vi "Get Network Adapter Settings.vi"(8 "error in":errorcluster, 11 "Refnum in":refnum<k21>) -> (0 "error out":errorcluster, 2 "Network Adapter Settings":T1[](array[typedef]) {"IP Address Request Mode" items=["Static"=1, "DHCP/Link Local"=2, "Link-Local Only"=4, "DHCP Only"=8]; "Adapter Type" items=["Ethernet"=1, "WLAN"=2]; "Adapter Mode" items=["Disabled"=1, "TCP/IP Ethernet"=2, "Deterministic"=4, "EtherCAT"=8, "TCP/IP WLAN Connect"=32, "TCP/IP WLAN Create"=64]}, 3 "Refnum out":refnum<k21>)   [LabVIEW 2015, in "RT Management.lvlib"]
uses:
  RT Management.lvlib
  Distributed Devices/Controls/NetworkAdapterSettings.ctl
  <vilib>/nisyscfg/Find Hardware.vi
  <vilib>/nisyscfg/Close (Hardware).vi
  <vilib>/nisyscfg/nisyscfg.lvlib
  <resource>/objmgr/niflexriosae.rc
  Distributed Devices/Device.lvclass
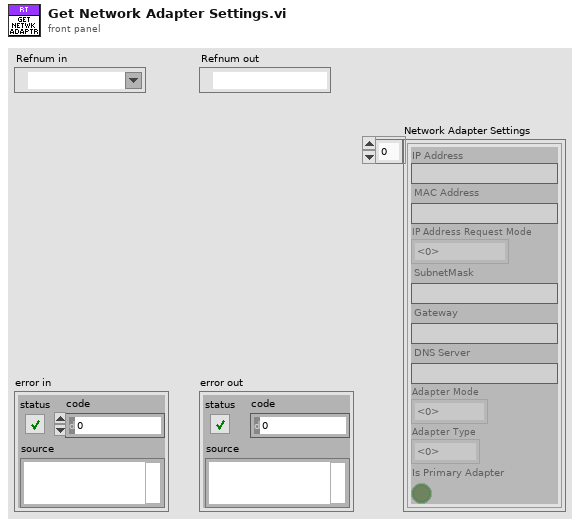
[diagram p1: front panel]
types:
  T1 = typedef "RT Management.lvlib/Device.lvclass/NetworkAdapterSettings.ctl" = cluster{"IP Address":string, "MAC Address":string, "IP Address Request Mode":u32, "SubnetMask":string, "Gateway":string, "DNS Server":string, "Adapter Mode":u32, "Adapter Type":u32, "Is Primary Adapter":bool}
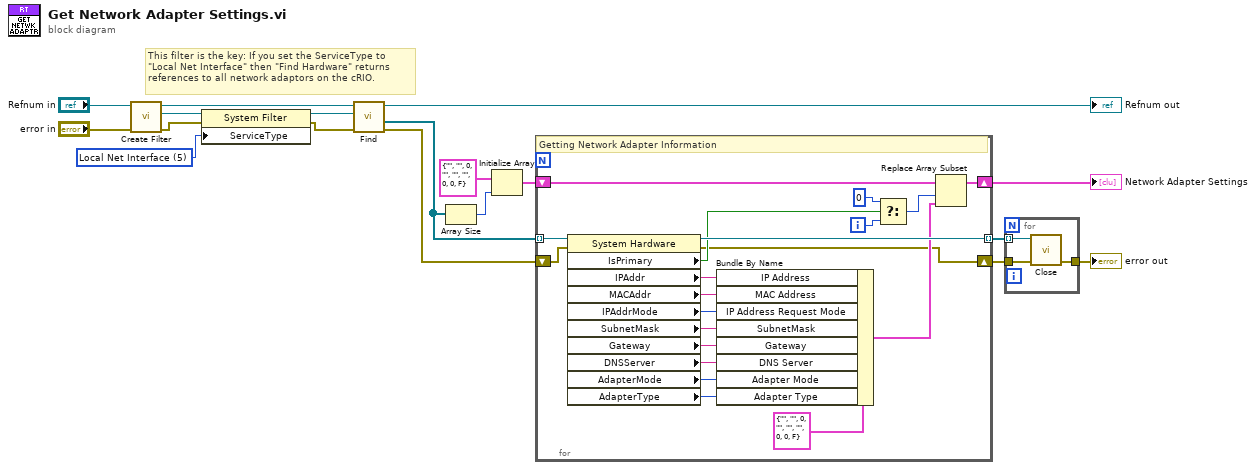
[diagram p0: block diagram]
diagram:
  w10 = u32 5 items=["NI Network Resource", "NI Real-Time", "NI System Configuration", "NI Web Interface", "Local System", "Local Net Interface", "Local Time Keeper", "Local Time Reference", "LXI Instrument"] ("Service Type")
  # "This filter is the key: If you set the ServiceType to\n\"Local Net Interface\" then \"Find Hardware\" returns\nreferences to all network adaptors on the cRIO."
  n1 = call <vilib>:"Create Filter.vi"("error in (no error)"="error in", "Session in"="Refnum in") -> ("error out"=w13:errorcluster, "Filter out"=w9:refnum<k20>, "Session out"=w8:refnum<k21>)  [unwired: 7 in]
  n2 = property class="System Filter"(reference=w9, error in=w13, "ServiceType"=w10) -> (reference out=w11:refnum<k20>, error out=w12:errorcluster)
  n3 = call-poly <vilib>:"Find.vi"("error in (no error)"=w12, "Filter in"=w11, "Session in"=w8) -> ("error out"=w14:errorcluster, "Resources out"=w4:refnum<k20>[], "Session out"=→"Refnum out":refnum<k21>)  [unwired: 5 in, 1 out]
  n4 = Array Size(array=w4) -> (size(s)=w3:i32)
  n5 = Initialize Array(T1 {"IP Address"="", "MAC Address"="", "IP Address Request Mode"=0, "SubnetMask"="", "Gateway"="", "DNS Server"="", "Adapter Mode"=0, "Adapter Type"=0, "Is Primary Adapter"=FALSE} ("Network Adapter Settings"), w3) -> (w1:T1[])
  n6 = for {
    tunnel: w4 -> [w37] mode=indexing
    shift-right: [w19] -> w17
    shift-left: w14 -> [w38]
    tunnel: [w32] -> w7 mode=indexing
    shift-right: [w20] -> w18
    shift-left: w1 -> [w26]
    i -> [w23]
    # "Getting Network Adapter Information"
    n7 = property class="System Hardware"(reference=w37, error in=w38) -> (reference out=w32:refnum<k20>, error out=w19:errorcluster, "IsPrimary"=w25:bool, "IPAddr"=w27:string, "MACAddr"=w33:string, "IPAddrMode"=w30:u32, "SubnetMask"=w34:string, "Gateway"=w35:string, "DNSServer"=w36:string, "AdapterMode"=w29:u32, "AdapterType"=w28:u32)
    n8 = Bundle By Name(cluster=T1 {"IP Address"="", "MAC Address"="", "IP Address Request Mode"=0, "SubnetMask"="", "Gateway"="", "DNS Server"="", "Adapter Mode"=0, "Adapter Type"=0, "Is Primary Adapter"=FALSE} ("Network Adapter Settings"), "IP Address"=w27, "MAC Address"=w33, "IP Address Request Mode"=w30, "SubnetMask"=w34, "Gateway"=w35, "DNS Server"=w36, "Adapter Mode"=w29, "Adapter Type"=w28) -> (w21:T1)
    n9 = Select(t=0 ("index"), s=w25, f=w23) -> (s? t:f=w22:i32)
    n10 = Replace Array Subset(array=w26, new element=w21, index=w22) -> (w20:T1[])
  }
  "Network Adapter Settings" <- w18
  n11 = for {
    tunnel: [w41] -> w16
    tunnel: w17 -> [w40]
    tunnel: w7 -> [w39] mode=indexing
    n12 = call-poly <vilib>:"Close.vi"("error in (no error)"=w40, "Resource in"=w39) -> ("error out"=w41:errorcluster)  [unwired: 9 in]
  }
  "error out" <- w16
